vi "GenerateCode.vi"(1 "Terms":T1[](array[typedef]), 3 "Diagram":refnum<vi>, 5 "XRef":refnum<vi>, 6 "State In":T4) -> (0 "Generated Code?":bool, 2 "State Out":T4, 4 "Reply":string[](array[string]))   [LabVIEW 2015, in "Control-Refs.xnode"]
doc: "This ability VI is called when it is time to define the execution behavior of your XNode via LabVIEW's scripting API. This VI is only called when you have previously informed LabVIEW that you need to script through a GenerateCode reply. Diagram is a reference to a diagram of a temporary VI. This diagram contains exactly one front panel terminal for each terminal of your XNode. Terms is an array of pairs of Term IDs and terminal references. LabVIEW will copy code scripted into this diagram into your XNode and connect everything to the correct terminals. The front panel terminals that are on this diagram are special in that they can only be on the top level diagram.\n \n Generate Code? is used to tell LabVIEW whether or not you want to copy the scripted diagram over. If there is an error and you wish not to commit the changes, then the old XNode behavior will be left unchanged. If you set Generate Code? to false, then this VI will be called again next time type propagation is run. Otherwise, it will not be called until you indicate that it should be through the reply on another ability VI.\n \n Because the diagram you are scripting into is separate from the VI containing the XNode instance, type propagation and the data manager will run on the temporary VI after each scripting call.\n \n You should not use the Copy scripting method to move code into the temporary VI. This will adversely affect the user's clipboard. You should use the Move scripting method instead.\n\nDefault behavior: None.\n\nThis ability does not provide UI and OS messages are not handled.\n\nSee also: ModifyCode"
uses:
  Control-Refs.xnode
  State.ctl
  <vilib>/XNodeSupport/XNodeTermIDPair.ctl
  <vilib>/XNodeSupport/XNodeTermRef.ctl
  <vilib>/XNodeSupport/XNodeString.ctl
  <vilib>/LV-Scripting/LV-Scripting.lvlib
  <vilib>/Utility/Data Type/NI_Data Type.lvlib
  <vilib>/XNodeSupport/NI_XNodeSupport.lvlib
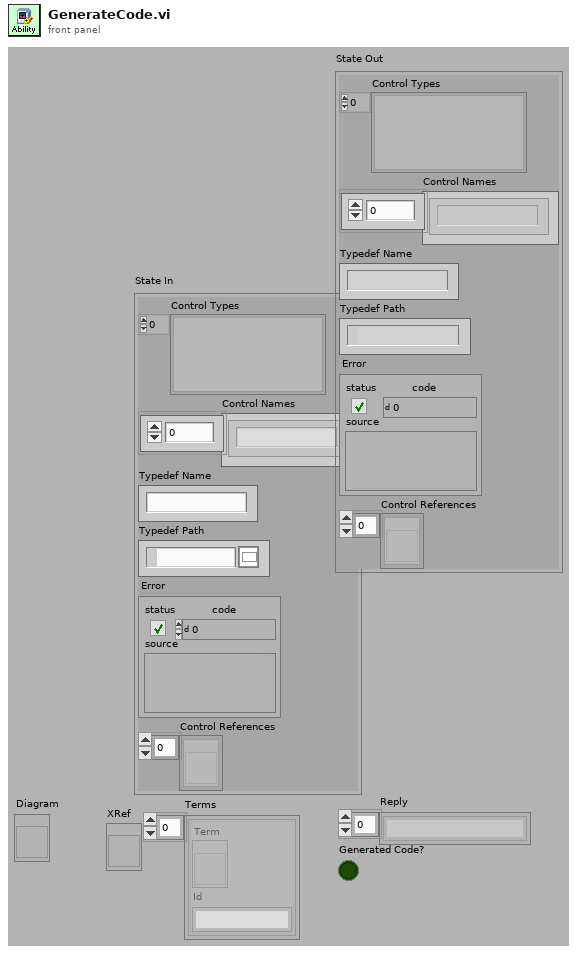
[diagram p1: front panel]
types:
  T1 = typedef "NI_XNodeSupport.lvlib/XNodeTermIDPair.ctl" = cluster{"Term":T2, "Id":T3}
  T2 = typedef "NI_XNodeSupport.lvlib/XNodeTermRef.ctl" = refnum<vi>
  T3 = typedef "NI_XNodeSupport.lvlib/XNodeString.ctl" = string
  T4 = typedef "Control-Refs.xnode/State.ctl" = cluster{"Control Types":variant[], "Control Names":string[], "Typedef Name":string, "Typedef Path":path, "Error":errorcluster, "Control References":refnum<vi>[]}
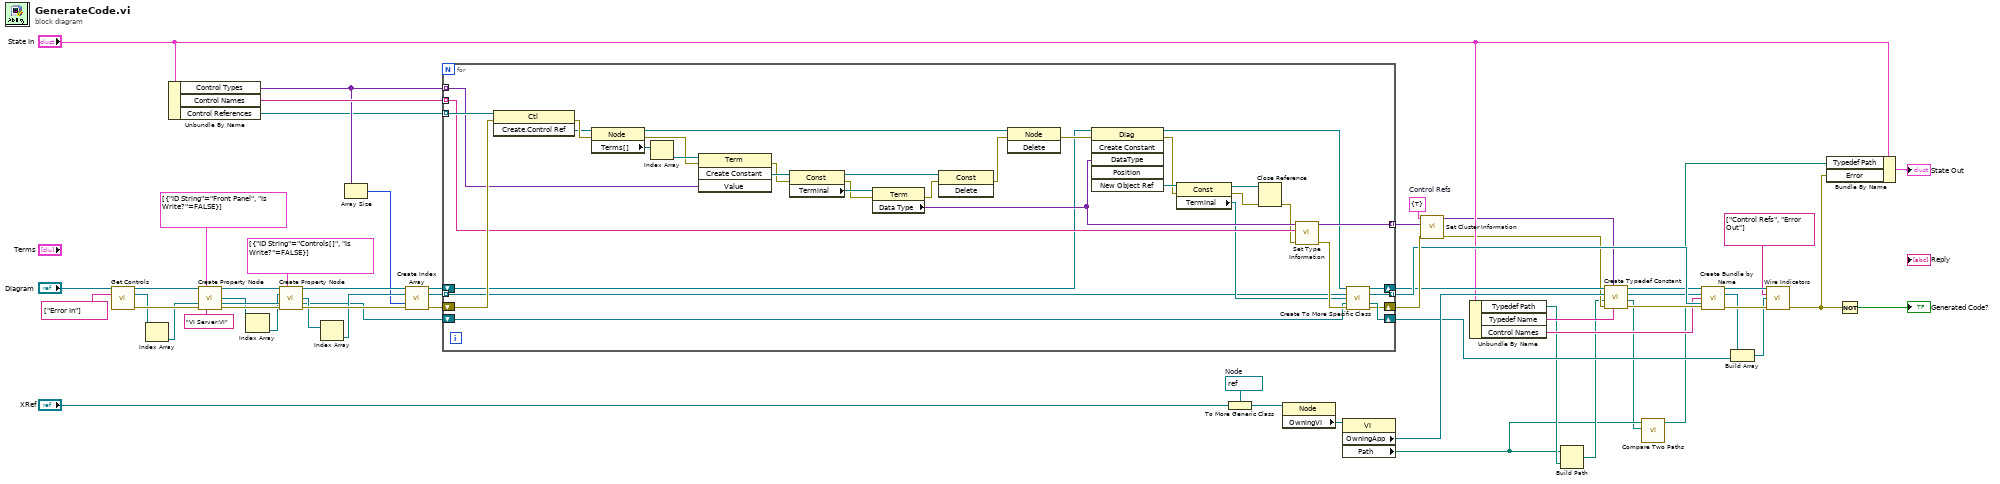
[diagram p0: block diagram]
diagram:
  w29 = refnum<vi> refnum  # Node
  w34 = cluster{bool} {TRUE}  # Control Refs
  n1 = call <vilib>:"Get Controls.vi"("Diagram in"="Diagram", "Control Names"=string[] ["Error In"]) -> ("Diagram out"=w56:refnum<vi>, "Control Terminals"=w50:refnum<vi>[], "error out"=w53:errorcluster)  [unwired: 11 in]
  n2 = Index Array(array=w50) -> (element=w47:refnum<vi>)  [unwired: 1 in]
  n3 = Unbundle By Name("State In") -> ("Control Types"=w41:variant[], "Control Names"=w42:string[], "Control References"=w35:refnum<vi>[])
  n4 = call <vilib>:"Create Property Node.vi"("Diagram in"=w56, "Properties"=cluster{"ID String":string, "Is Write?":bool}[] [{"ID String"="Front Panel", "Is Write?"=FALSE}], "error in"=w47, "error in (no error)"=w53, "Class Name"="VI Server:VI") -> ("Diagram out"=w55:refnum<vi>, "Outputs"=w18:refnum<vi>[], 10:"error out"=w38:refnum<vi>, 15:"error out"=w52:errorcluster)  [unwired: 6 in, 1 out]
  n5 = Index Array(array=w18) -> (element=w17:refnum<vi>)  [unwired: 1 in]
  n6 = call <vilib>:"Create Property Node.vi"("Diagram in"=w55, "Properties"=cluster{"ID String":string, "Is Write?":bool}[] [{"ID String"="Controls[]", "Is Write?"=FALSE}], "reference"=w17, "error in"=w38, "error in (no error)"=w52) -> ("Diagram out"=w54:refnum<vi>, "Outputs"=w45:refnum<vi>[], 10:"error out"=w37:refnum<vi>, 15:"error out"=w51:errorcluster)  [unwired: 6 in, 1 out]
  n7 = Index Array(array=w45) -> (element=w44:refnum<vi>)  [unwired: 1 in]
  n8 = Array Size(array=w41) -> (size(s)=w43:i32)
  n9 = call <vilib>:"Create Index Array.vi"("Diagram in"=w54, "array"=w44, "Index Count"=w43, "error in (no error)"=w51) -> ("Diagram out"=w39:refnum<vi>, "Outputs"=w40:refnum<vi>[], "error out"=w36:errorcluster)  [unwired: 9 in]
  n10 = for {
    tunnel: w42 -> [w72] mode=indexing
    tunnel: w41 -> [w59] mode=indexing
    tunnel: w40 -> [w68] mode=indexing
    shift-right: [w64] -> w16
    shift-left: w39 -> [w61]
    shift-right: [w66] -> w11
    shift-left: w37 -> [w67]
    shift-right: [w65] -> w32
    shift-left: w36 -> [w76]
    tunnel: w35 -> [w77] mode=indexing
    tunnel: [w63] -> w19 mode=indexing
    tunnel: [w62] -> w33 mode=indexing
    n11 = invoke class="Ctl" method="Create.Control Ref"(reference=w77, error in=w76) -> (error out=w90:errorcluster, "Create Control Ref"=w88:refnum<vi>)  [unwired: 1 in, 1 out]
    n12 = property class="Node"(reference=w88, error in=w90) -> (reference out=w91:refnum<vi>, error out=w89:errorcluster, "Terms[]"=w93:refnum<vi>[])
    n13 = Index Array(array=w93) -> (element=w92:refnum<vi>)  [unwired: 1 in]
    n14 = invoke class="Term" method="Create Constant"(reference=w92, error in=w89, "Value"=w59) -> (error out=w84:errorcluster, "Create Constant"=w85:refnum<vi>)  [unwired: 1 in, 2 out]
    n15 = property class="Const"(reference=w85, error in=w84) -> (reference out=w80:refnum<vi>, error out=w86:errorcluster, "Terminal"=w87:refnum<vi>)
    n16 = property class="Term"(reference=w87, error in=w86) -> (error out=w79:errorcluster, "Data Type"=w73:variant)  [unwired: 1 out]
    n17 = invoke class="Const" method="Delete"(reference=w80, error in=w79) -> (error out=w78:errorcluster)  [unwired: 1 in, 2 out]
    n18 = invoke class="Node" method="Delete"(reference=w91, error in=w78) -> (error out=w81:errorcluster)  [unwired: 1 in, 2 out]
    n19 = invoke class="Diag" method="Create Constant"(reference=w61, error in=w81, "DataType"=w73) -> (reference out=w60:refnum<vi>, error out=w82:errorcluster, "New Object Ref"=w83:refnum<vi>)  [unwired: 3 in, 3 out]
    n20 = property class="Const"(reference=w83, error in=w82) -> (reference out=w74:refnum<vi>, error out=w75:errorcluster, "Terminal"=w69:refnum<vi>)
    n21 = Close Reference(reference=w74, error in (no error)=w75) -> (error out=w71:errorcluster)
    n22 = call <vilib>:"Set Type Information.vi"("error in (no error)"=w71, "Name"=w72, "Variant in"=w73) -> ("error out"=w70:errorcluster, "Variant out"=w62:variant)  [unwired: 7 in]
    n23 = call <vilib>:"Create To More Specific Class.vi"("Diagram in"=w60, "reference"=w68, "target class"=w69, "error in"=w67, "error in (no error)"=w70) -> ("Diagram out"=w64:refnum<vi>, "specific class reference"=w63:refnum<vi>, 10:"error out"=w66:refnum<vi>, 15:"error out"=w65:errorcluster)  [unwired: 7 in]
  }
  n24 = To More Generic Class(target class=w29, reference="XRef") -> (generic class reference=w30:refnum<vi>)
  n25 = property class="Node"(reference=w30) -> ("OwningVI"=w28:refnum<vi>)  [unwired: 1 in, 2 out]
  n26 = property class="VI"(reference=w28) -> ("OwningApp"=w15:refnum<vi>, "Path"=w3:path)  [unwired: 1 in, 2 out]
  n27 = call <vilib>:"Set Cluster Information.vi"("error in (no error)"=w32, "Cluster Elements"=w33, "Variant in"=w34) -> ("error out"=w12:errorcluster, "Variant out"=w7:variant)  [unwired: 7 in]
  n28 = Unbundle By Name("State In") -> ("Typedef Path"=w5:path, "Typedef Name"=w13:string, "Control Names"=w6:string[])
  n29 = Build Path(base path=w3, name or relative path=w5) -> (appended path=w4:path)
  n30 = call <vilib>:"Create Typedef Constant.vi"("Typedef Name"=w13, "Type"=w7, "error in (no error)"=w12, "Typedef Path"=w4, "Application"=w15, "Diagram in"=w16) -> ("error out"=w10:errorcluster, "New Typedef Path"=w2:path, "Constant"=w8:refnum<vi>, "Diagram out"=w9:refnum<vi>)  [unwired: 2 in]
  n31 = call <vilib>:"Compare Two Paths.vi"("Path 2"=w2, "Path 1"=w3) -> ("Relative Path from 1 to 2"=w1:path)  [unwired: 6 in, 3 out]
  n32 = call <vilib>:"Create Bundle by Name.vi"("Diagram in"=w9, "input cluster"=w8, "Element Names"=w6, "Inputs"=w19, "error in (no error)"=w10) -> ("Diagram out"=w27:refnum<vi>, "output cluster"=w25:refnum<vi>, "error out"=w26:errorcluster)  [unwired: 8 in]
  n33 = Build Array(w25, w11) -> (w24:refnum<vi>[])
  n34 = call <vilib>:"Wire Indicators.vi"("Diagram in"=w27, "Indicator Names"=string[] ["Control Refs", "Error Out"], "Outputs"=w24, "error in (no error)"=w26) -> ("error out"=w21:errorcluster)  [unwired: 10 in, 1 out]
  n35 = Bundle By Name(cluster="State In", "Typedef Path"=w1, "Error"=w21) -> (→"State Out":T4)
  n36 = Not(x=w21) -> (.not. x?=→"Generated Code?":bool)
